vi "UserLED_Toggle.vi"(2 "Player":u8) -> ()   [LabVIEW 2018]
uses:
  <vilib>/rvi/eio/common/nirviEmuTemplateMethod_errors.vi
  <vilib>/eio/EIONode/EIONode.xnode
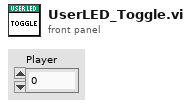
[diagram p1: front panel]
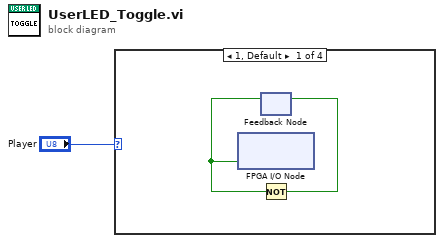
[diagram p0: block diagram]
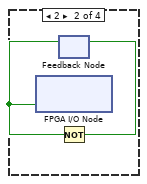
[diagram p2: hidden frame]
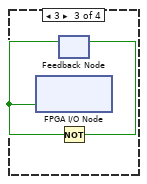
[diagram p3: hidden frame]
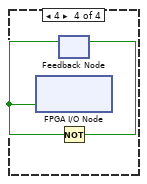
[diagram p4: hidden frame]
diagram:
  n1 = case shown="1, Default" "Player" {
    frame 1, Default {
      n2 = feedback #1() -> (w2:bool)  [unwired: 1 in]
      n3 = xnode "FPGA I/O Node"("LED0"=w2) -> ()  [unwired: 1 in, 1 out]
      n4 = Not(x=w2) -> (.not. x?=w3:bool)
      n5 = feedback-in #1(w3) -> ()
    }
    frame 2 {
      n6 = feedback #2() -> (w4:bool)  [unwired: 1 in]
      n7 = xnode "FPGA I/O Node"("LED1"=w4) -> ()  [unwired: 1 in, 1 out]
      n8 = Not(x=w4) -> (.not. x?=w5:bool)
      n9 = feedback-in #2(w5) -> ()
    }
    frame 3 {
      n10 = feedback #3() -> (w6:bool)  [unwired: 1 in]
      n11 = xnode "FPGA I/O Node"("LED2"=w6) -> ()  [unwired: 1 in, 1 out]
      n12 = Not(x=w6) -> (.not. x?=w7:bool)
      n13 = feedback-in #3(w7) -> ()
    }
    frame 4 {
      n14 = feedback #4() -> (w8:bool)  [unwired: 1 in]
      n15 = xnode "FPGA I/O Node"("LED3"=w8) -> ()  [unwired: 1 in, 1 out]
      n16 = Not(x=w8) -> (.not. x?=w9:bool)
      n17 = feedback-in #4(w9) -> ()
    }
  }
